vi "EditPolyVI.vi"() -> ()   [LabVIEW 2016]
uses:
  src/main/apis/Stimulus/Stimulus [Poly].vi
  src/main/Drona.lvlib
panel:
  in  "Set(T)/Get(F)":bool
  in  "InstanceInfo 2":T1(array[cluster])
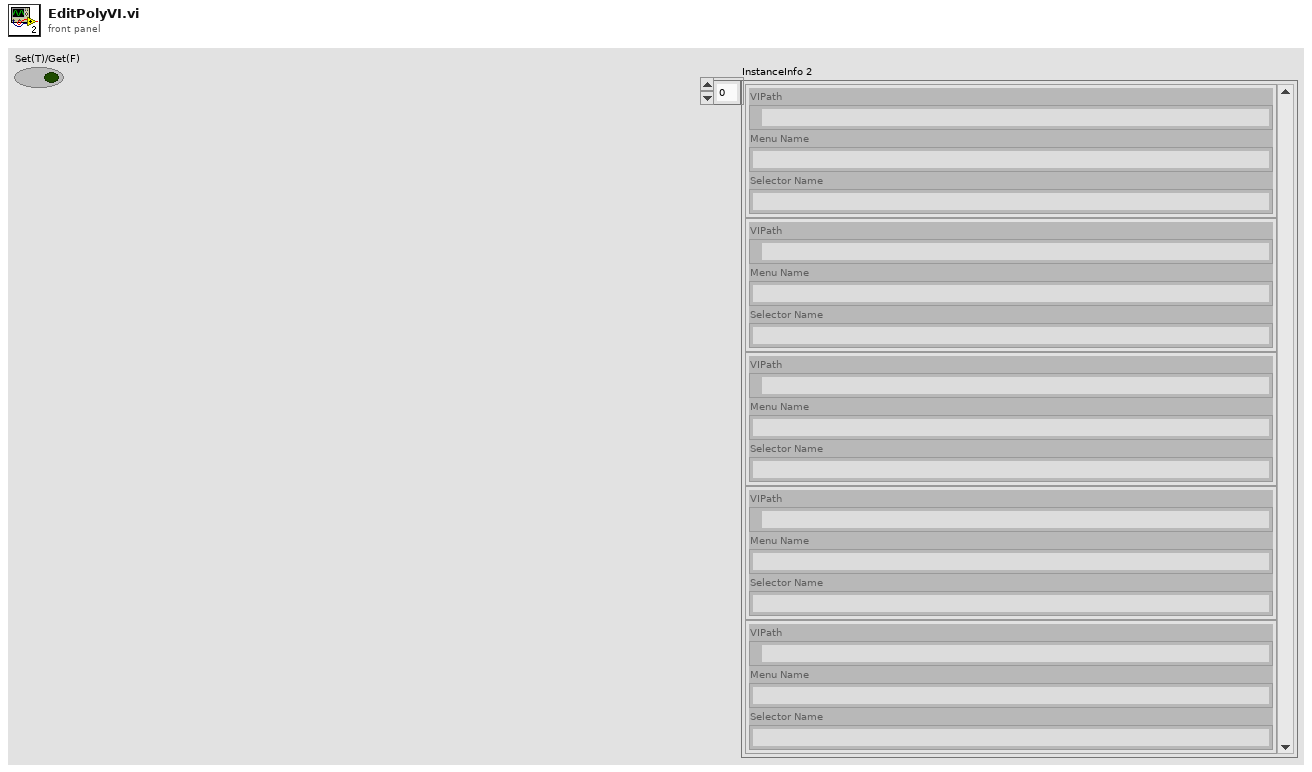
[diagram p1: front panel]
types:
  T1 = cluster{"VIPath":path, "Menu Name":string, "Selector Name":string}[]
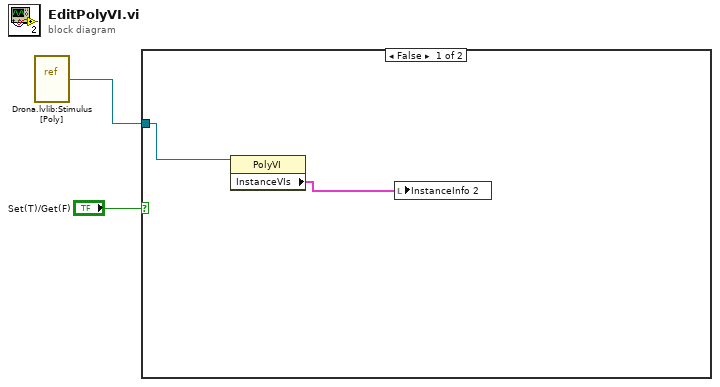
[diagram p0: block diagram]
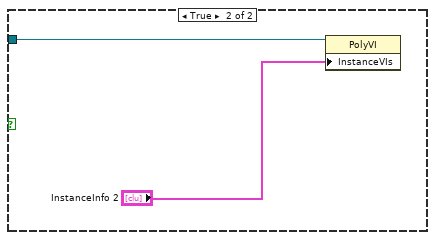
[diagram p2: hidden frame]
diagram:
  n1 = vi-ref "Drona.lvlib:Stimulus [Poly].vi"() -> (w2:refnum<vi>)
  n2 = case shown="False" "Set(T)/Get(F)" {
    tunnel: w2 -> [w4 w5]
    frame False {
      n3 = property class="PolyVI"(reference=w4) -> ("InstanceVIs"=w3:T1)  [unwired: 1 in, 2 out]
      n4 = local write "InstanceInfo 2"(w3) -> ()
    }
    frame True {
      n5 = property class="PolyVI"(reference=w5, "InstanceVIs"="InstanceInfo 2") -> ()  [unwired: 1 in, 2 out]
    }
  }
